vi "Convert Pulse Width to Distance.vi"(11 "pulse width (uSec)":u32) -> (3 "distance (m)":fxp<+,32,8> format="%.27g")   [LabVIEW 2013, in "NI_Robotics_Parallax PING))) (FPGA).lvlib"]
doc: "Converts the pulse width to distance in m."
uses:
  NI_Robotics_Parallax PING))) (FPGA).lvlib
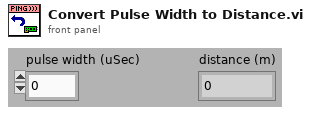
[diagram p1: front panel]
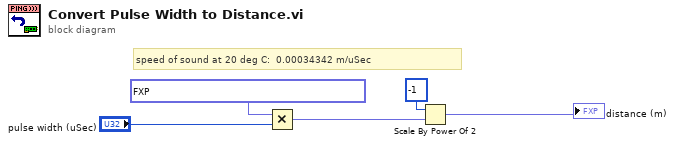
[diagram p0: block diagram]
diagram:
  # "speed of sound at 20 deg C:  0.00034342 m/uSec"
  n1 = Multiply(x=fxp<+,18,-11> 0.00034341961145401 ("y"), y="pulse width (uSec)") -> (x*y=w4:fxp<+,32,8>)
  n2 = Scale By Power Of 2(n=-1, x=w4) -> (x*2^n=→"distance (m)":fxp<+,32,8>)
